vi "Update Names Array.vi"(7 "index of element":i32, 9 "Assert Data":string, 11 "Assert List in":string[](array[string])) -> (3 "Assert List out":string[](array[string]))   [LabVIEW 2016, in "AssertEngine.lvlib" / "AssertEngine.lvclass"]
doc: "Updates the string array of assert names, either by adding a new element or leaving the array as it is (if the item is present it doesn't need to be replaced)"
uses:
  AssertEngine.lvclass
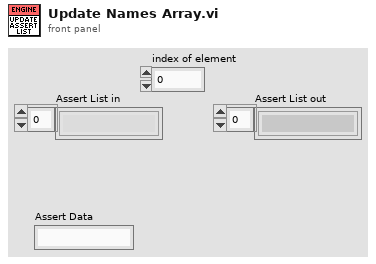
[diagram p1: front panel]
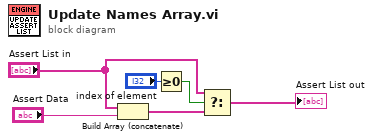
[diagram p0: block diagram]
diagram:
  n1 = Build Array (concatenate)("Assert List in", "Assert Data") -> (w4:string[])
  n2 = Greater Or Equal To 0?(x="index of element") -> (x >= 0?=w1:bool)
  n3 = Select(t="Assert List in", s=w1, f=w4) -> (s? t:f=→"Assert List out":string[])
